vi "controlFL.vi"() -> ()   [LabVIEW 2021]
panel:
  out "Control":T1(graph)
  out "X2 2":dynamicdata(graph)
  out "X1 2":dynamicdata(graph)
  out "SeñalU":cluster{"X":dbl[], "Y":dbl[]}[](graph)
  out "Error":cluster{"X":dbl[], "Y":dbl[]}[](graph)
  in  "stop":bool
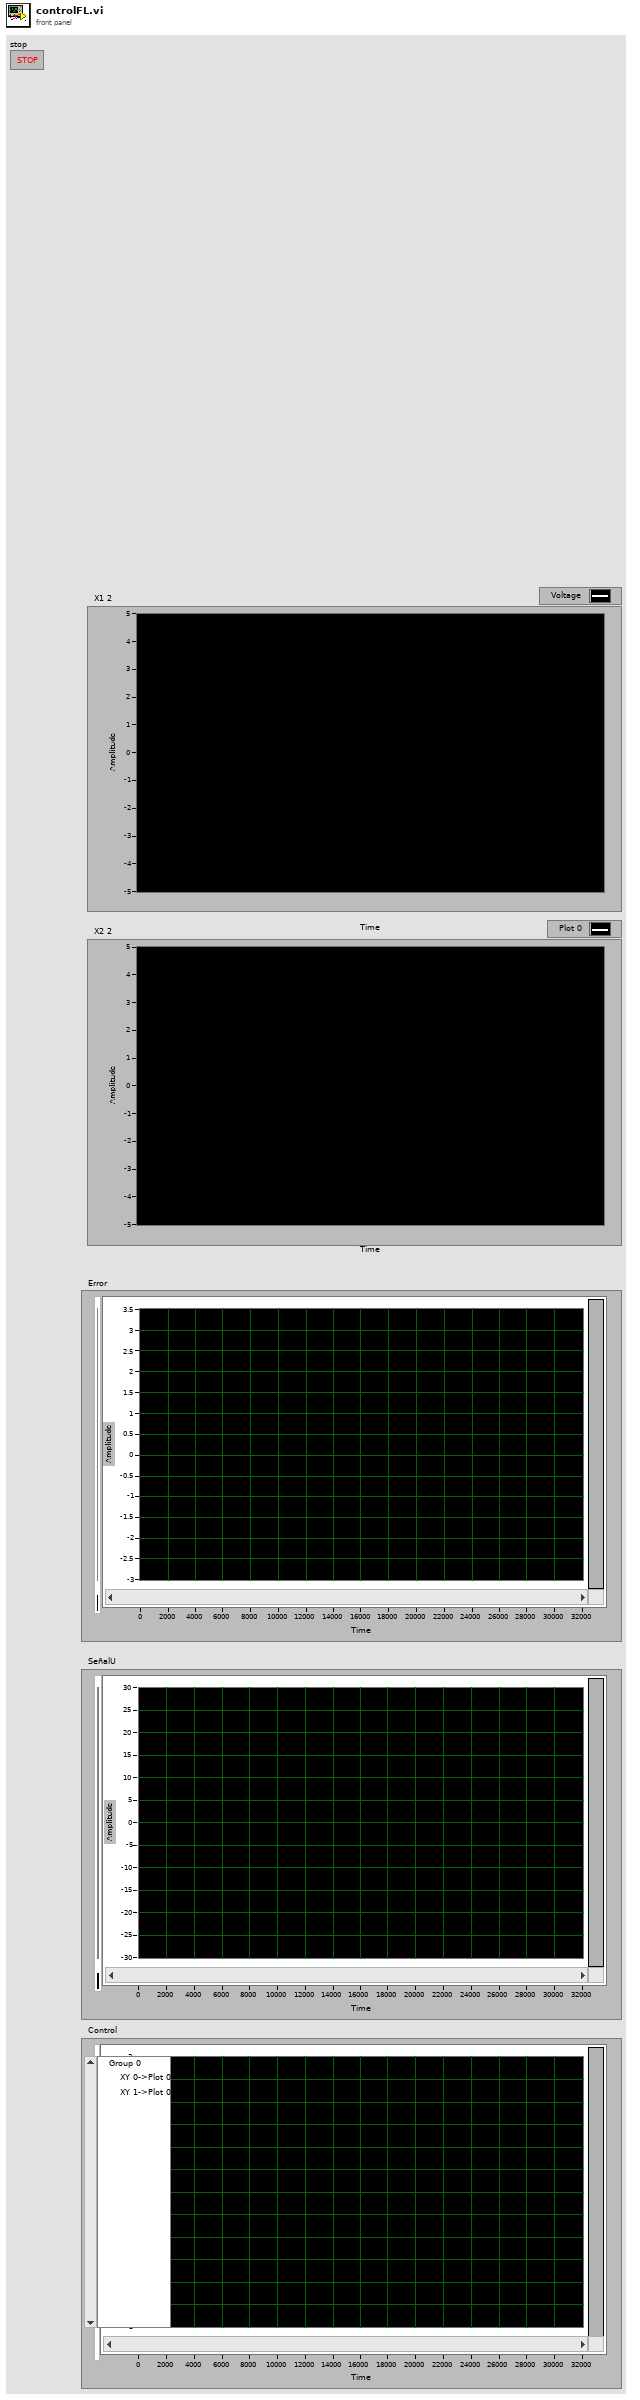
[diagram p1: front panel]
types:
  T1 = cluster{"XY Graph":cluster{"X":dbl[], "Y":dbl[]}[], "XY Graph":cluster{"X":dbl[], "Y":dbl[]}[]}
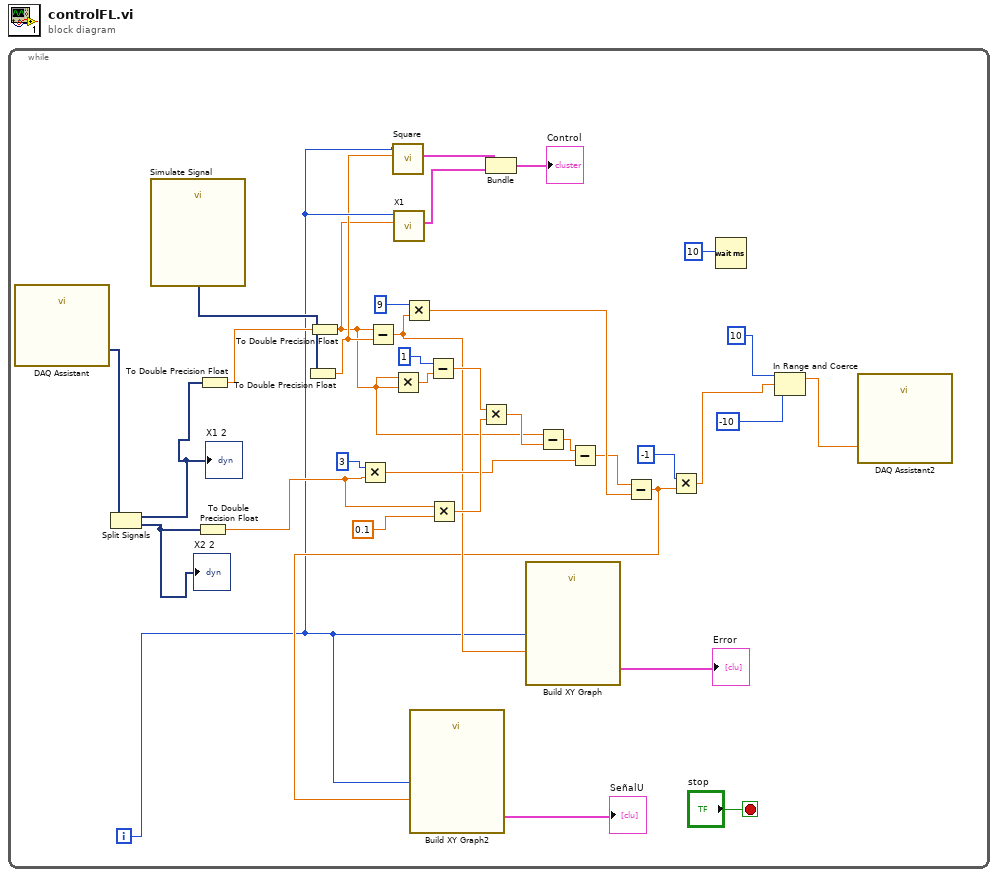
[diagram p0: block diagram]
diagram:
  n1 = while {
    i -> [w3]
    stop <- "stop" stop-if-true
    n2 = call "DAQ Assistant"() -> ("data"=w18:dynamicdata)  [unwired: 17 in, 2 out]
    n3 = Split Signals(w18) -> (w16:dynamicdata, w17:dynamicdata)  [unwired: 2 in]
    "X1 2" <- w16
    "X2 2" <- w17
    n4 = call "Simulate Signal"() -> ("Square"=w7:dynamicdata)  [unwired: 14 in, 1 out]
    n5 = To Double Precision Float(number=w17) -> (double precision float=w14:dbl)
    n6 = To Double Precision Float(number=w16) -> (double precision float=w15:dbl)
    n7 = To Double Precision Float(number=w7) -> (double precision float=w2:dbl)
    n8 = To Double Precision Float(number=w15) -> (double precision float=w1:dbl)
    n9 = Multiply(x=3, y=w14) -> (x*y=w24:dbl)
    n10 = Subtract(x=w1, y=w2) -> (x-y=w21:dbl)
    n11 = call "Square"("Y Input"=w2, "X Input"=w3) -> ("XY Graph"=w4:cluster{"X":dbl[], "Y":dbl[]}[])  [unwired: 8 in, 1 out]
    n12 = Multiply(x=w1, y=w1) -> (x*y=w27:dbl)
    n13 = call "X1"("Y Input"=w1, "X Input"=w3) -> ("XY Graph"=w5:cluster{"X":dbl[], "Y":dbl[]}[])  [unwired: 8 in, 1 out]
    n14 = Multiply(x=9, y=w21) -> (x*y=w23:dbl)
    n15 = Subtract(x=1, y=w27) -> (x-y=w26:dbl)
    n16 = Multiply(x=w14, y=0.1) -> (x*y=w25:dbl)
    n17 = Multiply(x=w26, y=w25) -> (x*y=w9:dbl)
    n18 = Bundle("XY Graph"=w4, "XY Graph"=w5) -> (→"Control":T1)  [unwired: 1 in]
    n19 = call "Build XY Graph"("Y Input"=w21, "X Input"=w3) -> ("XY Graph"=→"Error":cluster{"X":dbl[], "Y":dbl[]}[])  [unwired: 8 in, 1 out]
    n20 = Subtract(x=w1, y=w9) -> (x-y=w8:dbl)
    n21 = Subtract(x=w8, y=w24) -> (x-y=w22:dbl)
    n22 = Subtract(x=w22, y=w23) -> (x-y=w20:dbl)
    n23 = call "Build XY Graph2"("Y Input"=w20, "X Input"=w3) -> ("XY Graph"=→"SeñalU":cluster{"X":dbl[], "Y":dbl[]}[])  [unwired: 8 in, 1 out]
    n24 = Multiply(x=-1, y=w20) -> (x*y=w11:dbl)
    n25 = Wait (ms)(milliseconds to wait=10) -> ()  [unwired: 1 out]
    n26 = In Range and Coerce(upper limit=10, x=w11, lower limit=-10) -> (coerced(x)=w10:dbl)  [unwired: 1 out]
    n27 = call "DAQ Assistant2"("data"=w10) -> ()  [unwired: 17 in, 2 out]
  }
